vi "流程文件XML解析.vi"(5 "简易流程Id":u16(ring), 7 "是否是简易流程":bool, 10 "添加的路径":path, 11 "参数簇":T2={"启动参数"=1, "启动模式"=enum."跨度核查", "量程"=enum."低量程"} {"启动参数" items=["总磷"=1, "总氮"=2, "氨氮"=3]}) -> (3 "数组":T1(array[cluster]) {"port" format="%08x"})   [LabVIEW 2016, in "斯坦道CODCr.lvlib"]
uses:
  <vilib>/xml/Load XML File.vi
  <vilib>/xml/Close Reference(Node).vi
  <resource>/objmgr/DOMUserDefRef.rc
  <vilib>/xml/NI_XML.lvlib
panel:
  in  "数值":i32
  out "字符串":string
  out "大小":i32
  out "XML字符串":string="<?xml version=\"1.0\" encoding=\"ISO-8859-1\"?>\n<bookstore>\n<book ISBN=\"978-0545128285\">\n  <title lang=\"en\">The Tales of Beedle the Bard</title>\n  <author>J. K. Rowling</author>\n  <year>2008</year>\n  <price>12.99</price>\n</book>\n<book ISBN=\"978-0316160209\">\n  <title lang=\"en\">Eclipse</title>\n  <author>Stephenie Meyer</author>\n  <year>2007</year>\n  <price>19.99</price>\n</book>\n<book ISBN=\"978-0316067928\">\n  <title lang=\"en\">Breaking Dawn</title>\n  <author>Stephenie Meyer</author>\n  <year>2008</year>\n  <price>22.99</price>\n</book>\n<book ISBN=\"978-0316017923\">\n  <title lang=\"en\">Outliers: The Story of Success</title>\n  <author>Malcolm Gladwell</author>\n  <year>2008</year>\n  <price>27.99</price>\n</book>\n<book ISBN=\"978-0596007645\">\n  <title lang=\"en\">XML in a Nutshell</title>\n  <author>Elliotte Rusty Harold</author>\n  <author>W. Scott Means</author>\n  <year>2004</year>\n  <price>39.95</price>\n</book>\n</bookstore>"
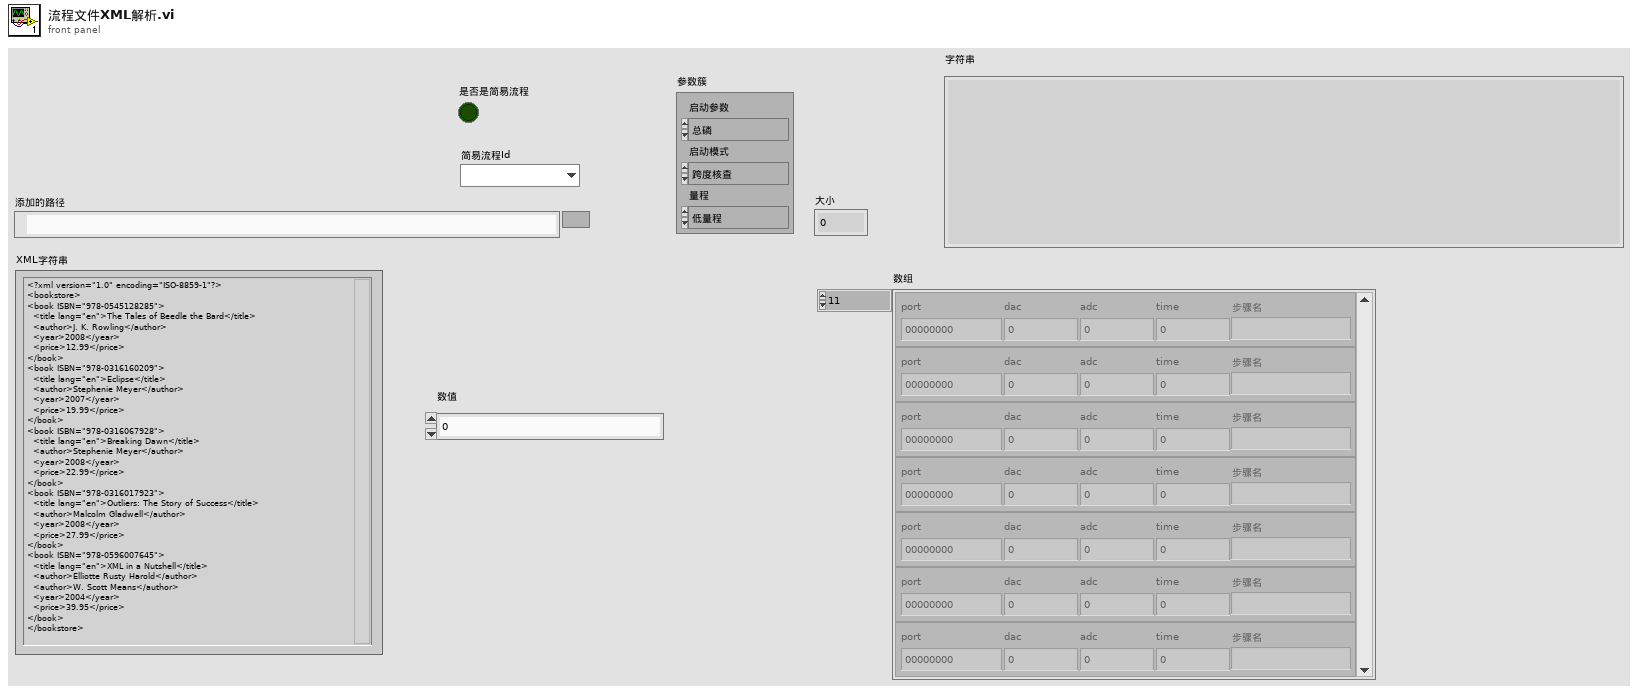
[diagram p1: front panel]
types:
  T1 = cluster{"port":i32, "dac":u8, "adc":u8, "time":u16, "步骤名":string}[]
  T2 = cluster{"启动参数":u16, "启动模式":enum16{"跨度核查", "水样测量", "零点核查", "标样核查", "加标回收", "快捷测试", "空白校准", "标样校准"}, "量程":enum16{"低量程", "高量程"}}
  T3 = enum16{"跨度核查", "水样测量", "零点核查", "标样核查", "加标回收", "快捷测试", "空白校准", "标样校准"}
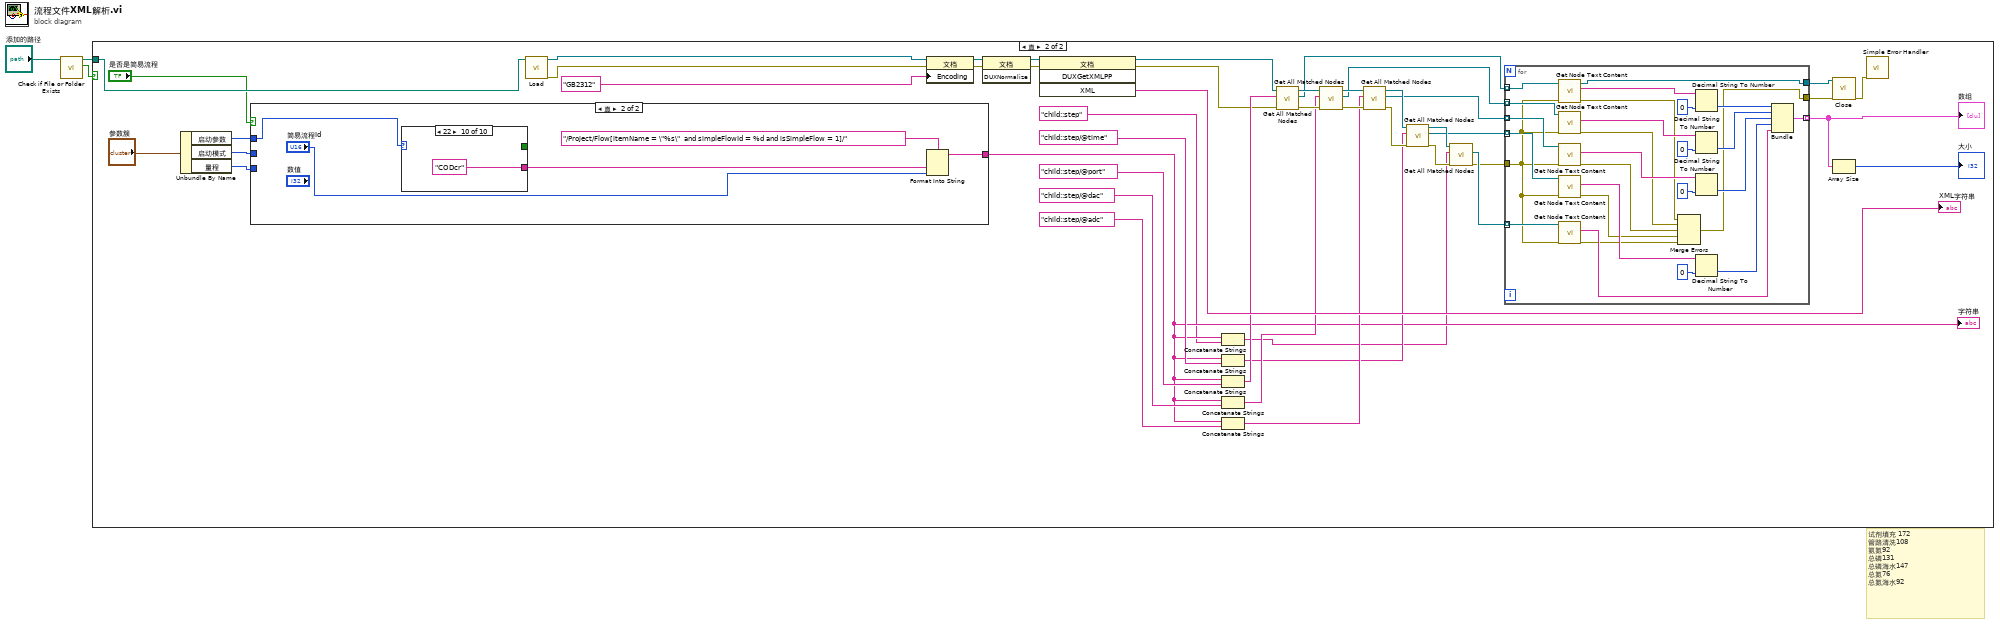
[diagram p0: block diagram]
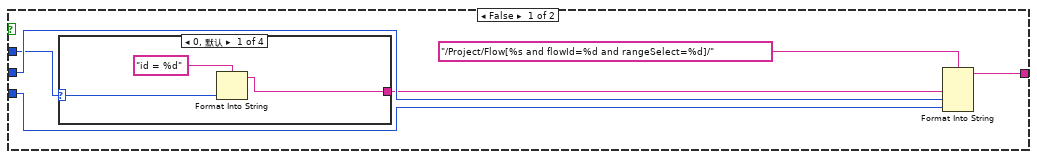
[diagram p3: hidden frame]
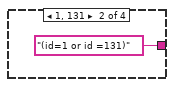
[diagram p4: hidden frame]
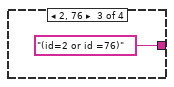
[diagram p5: hidden frame]
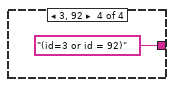
[diagram p6: hidden frame]
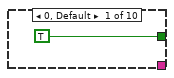
[diagram p7: hidden frame]
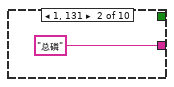
[diagram p8: hidden frame]
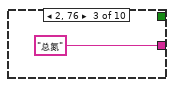
[diagram p9: hidden frame]
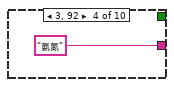
[diagram p10: hidden frame]
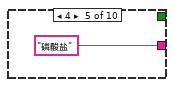
[diagram p11: hidden frame]
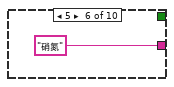
[diagram p12: hidden frame]
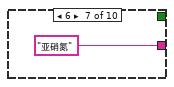
[diagram p13: hidden frame]
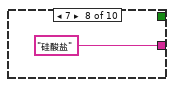
[diagram p14: hidden frame]
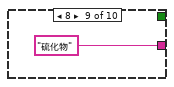
[diagram p15: hidden frame]
diagram:
  # "试剂填充 172 \n管路清洗108\n氨氮92\n总磷131\n总磷海水147\n总氮76\n总氮海水92"
  n1 = call <vilib>:"Check if File or Folder Exists.vi"("path"="添加的路径") -> ("file or folder exists?"=w1:bool, "dup path"=w2:path)  [unwired: 8 in, 1 out]
  n2 = case shown="真" w1 {
    tunnel: w2 -> [_ w35]
    frame False {
    }
    frame True {
      n3 = Unbundle By Name("参数簇") -> ("启动参数"=w36:u16, "启动模式"=w39:T3, "量程"=w38:enum16{"低量程", "高量程"})
      n4 = case shown="真" "是否是简易流程" {
        tunnel: w39 -> [w54 _]
        tunnel: w38 -> [w53 _]
        tunnel: w36 -> [w52 w63]
        tunnel: [w50 w65] -> w17
        frame False {
          n5 = case shown="0, 默认" w52 {
            selector: w52 -> [w57 _ _ _]
            tunnel: [w56 "(id=1 or id =131)" ("输入 4") "(id=2 or id =76)" ("输入 4") "(id=3 or id = 92)" ("输入 4")] -> w51
            frame 0, Default {
              n6 = Format Into String(format string="id = %d" ("格式字符串"), w57) -> (resulting string=w56:string)  [unwired: 2 in, 1 out]
            }
            frame 1, 131 {
            }
            frame 2, 76 {
            }
            frame 3, 92 {
            }
          }
          n7 = Format Into String(format string="/Project/Flow[%s and flowId=%d and rangeSelect=%d]/" ("XPath expression"), w51, w54, w53) -> (resulting string=w50:string)  [unwired: 2 in, 1 out]
        }
        frame True {
          n8 = case shown="22" w63 {
            tunnel: [_ "总磷" ("table输入") "总氮" ("table输入") "氨氮" ("table输入") "磷酸盐" ("table输入") "硝氮" ("table输入") "亚硝氮" ("table输入") "硅酸盐" ("table输入") "硫化物" ("table输入") "CODcr" ("table输入")] -> w62
            tunnel: [TRUE _ _ _ _ _ _ _ _ _] -> _
            frame 0, Default {
            }
            frame 1, 131 {
            }
            frame 2, 76 {
            }
            frame 3, 92 {
            }
            frame 4 {
            }
            frame 5 {
            }
            frame 6 {
            }
            frame 7 {
            }
            frame 8 {
            }
            frame 22 {
            }
          }
          n9 = Format Into String(format string="/Project/Flow[itemName = \"%s\"  and simpleFlowId = %d and isSimpleFlow = 1]/" ("XPath expression"), w62, "简易流程Id") -> (resulting string=w65:string)  [unwired: 2 in, 1 out]
        }
      }
      "字符串" <- w17
      n10 = call-poly <vilib>:"Load.vi"("path to XML document"=w35) -> ("DOM document out"=w47:refnum<k20>, "error out"=w46:errorcluster)  [unwired: 12 in, 1 out]
      n11 = property on="属性节点" class="文档"(reference=w47, error in=w46, "Encoding"="GB2312" ("文档编码")) -> (reference out=w45:refnum<k20>, error out=w44:errorcluster)
      n12 = invoke on="Invoke Node" class="文档" method="DUXNormalize"(reference=w45, error in=w44) -> (reference out=w42:refnum<k20>, error out=w43:errorcluster)  [unwired: 1 in, 1 out]
      n13 = invoke on="Invoke Node" class="文档" method="DUXGetXMLPP"(reference=w42, error in=w43) -> (reference out=w34:refnum<k20>, error out=w8:errorcluster, "XML"=→"XML字符串":string)  [unwired: 2 in, 1 out]
      n14 = Concatenate Strings(w17, "child::step" ("输入 4")) -> (w10:string)
      n15 = Concatenate Strings(w17, "child::step/@time" ("输入 4")) -> (w19:string)
      n16 = Concatenate Strings(w17, "child::step/@port" ("输入 4")) -> (w33:string)
      n17 = Concatenate Strings(w17, "child::step/@dac" ("输入 4")) -> (w23:string)
      n18 = Concatenate Strings(w17, "child::step/@adc" ("输入 4")) -> (w21:string)
      n19 = call <vilib>:"Get All Matched Nodes.vi"("error in (no error)"=w8, "XPath expression"=w33, "node in"=w34) -> ("error out"=w30:errorcluster, "node result array"=w15:refnum<k20>[], "node out"=w31:refnum<k20>)  [unwired: 6 in]
      n20 = call <vilib>:"Get All Matched Nodes.vi"("error in (no error)"=w30, "XPath expression"=w23, "node in"=w31) -> ("error out"=w29:errorcluster, "node result array"=w14:refnum<k20>[], "node out"=w28:refnum<k20>)  [unwired: 6 in]
      n21 = call <vilib>:"Get All Matched Nodes.vi"("error in (no error)"=w29, "XPath expression"=w21, "node in"=w28) -> ("error out"=w27:errorcluster, "node result array"=w13:refnum<k20>[], "node out"=w26:refnum<k20>)  [unwired: 6 in]
      n22 = call <vilib>:"Get All Matched Nodes.vi"("error in (no error)"=w27, "XPath expression"=w19, "node in"=w26) -> ("error out"=w25:errorcluster, "node result array"=w12:refnum<k20>[], "node out"=w24:refnum<k20>)  [unwired: 6 in]
      n23 = call <vilib>:"Get All Matched Nodes.vi"("error in (no error)"=w25, "XPath expression"=w10, "node in"=w24) -> ("error out"=w9:errorcluster, "node result array"=w11:refnum<k20>[])  [unwired: 6 in, 1 out]
      n24 = for {
        tunnel: w15 -> [w103] mode=indexing
        tunnel: w14 -> [w102] mode=indexing
        tunnel: w13 -> [w101] mode=indexing
        tunnel: w12 -> [w100] mode=indexing
        tunnel: w11 -> [w99] mode=indexing
        tunnel: [w85] -> w5 mode=indexing
        tunnel: w9 -> [w79]
        tunnel: [w78] -> w7
        tunnel: [w77] -> w6
        n25 = call <vilib>:"Get Node Text Content.vi"("error in (no error)"=w79, "node in"=w103) -> ("error out"=w84:errorcluster, "node text"=w98:string, "node out"=w77:refnum<k20>)  [unwired: 7 in]
        n26 = call <vilib>:"Get Node Text Content.vi"("error in (no error)"=w79, "node in"=w102) -> ("error out"=w83:errorcluster, "node text"=w95:string)  [unwired: 7 in, 1 out]
        n27 = call <vilib>:"Get Node Text Content.vi"("error in (no error)"=w79, "node in"=w101) -> ("error out"=w82:errorcluster, "node text"=w92:string)  [unwired: 7 in, 1 out]
        n28 = call <vilib>:"Get Node Text Content.vi"("error in (no error)"=w79, "node in"=w100) -> ("error out"=w81:errorcluster, "node text"=w91:string)  [unwired: 7 in, 1 out]
        n29 = call <vilib>:"Get Node Text Content.vi"("error in (no error)"=w79, "node in"=w99) -> ("error out"=w80:errorcluster, "node text"=w86:string)  [unwired: 7 in, 1 out]
        n30 = Merge Errors(w84, w83, w82, w81, w80) -> (w78:errorcluster)
        n31 = Decimal String To Number(string=w98, default (0L)=0 ("默认(0 I32)")) -> (number=w90:i32)  [unwired: 1 in, 1 out]
        n32 = Decimal String To Number(string=w95, default (0L)=u8 0 ("默认(0 I32)")) -> (number=w89:u8)  [unwired: 1 in, 1 out]
        n33 = Decimal String To Number(string=w92, default (0L)=u8 0 ("默认(0 I32)")) -> (number=w88:u8)  [unwired: 1 in, 1 out]
        n34 = Decimal String To Number(string=w91, default (0L)=u16 0 ("默认(0 I32)")) -> (number=w87:u16)  [unwired: 1 in, 1 out]
        n35 = Bundle(w90, w89, w88, w87, "node text"=w86) -> (w85:cluster{i32, u8, u8, u16, "node text":string})  [unwired: 1 in]
      }
      "数组" <- w5
      n36 = call-poly <vilib>:"Close.vi"("error in (no error)"=w7, "node"=w6) -> ("error out"=w41:errorcluster)  [unwired: 7 out]
      n37 = Array Size(array=w5) -> (size(s)=→"大小":i32)
      n38 = call <vilib>:"Simple Error Handler.vi"("error in (no error)"=w41) -> ()  [unwired: 4 in, 5 out]
    }
  }
